vi "iow28_io-ports_write.vi"() -> ()   [LabVIEW 2011]
panel:
  out "Error Read":errorcluster caption="error"
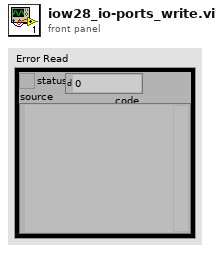
[diagram p1: front panel]
types:
  T1 = typedef "IOWarrior_Handle.ctl" = cluster{"Handle":u32, "Serial Number":string, "type of Warrior":T2, "Root Handle":bool, "Revision":u16}
  T2 = typedef "IOWarrior_Type.ctl" = enum16{"invalid", "IOW24", "IOW40", "IOW56", "IOPV1", "IOPV2", "IOW28"}
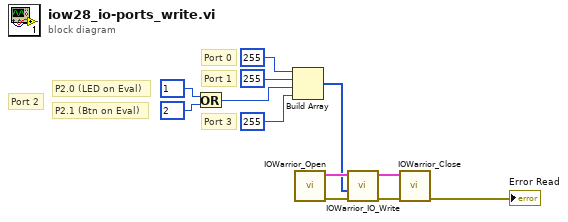
[diagram p0: block diagram]
diagram:
  # "Port 2"
  # "P2.1 (Btn on Eval)"
  # "Port 3"
  # "P2.0 (LED on Eval)"
  # "Port 1"
  # "Port 0"
  n1 = Or(x=u8 1, y=u8 2) -> (x .or. y?=w1:u8)
  n2 = Build Array(u8 255, u8 255, w1, u8 255) -> (w7:u8[])
  n3 = call "IOWarrior_Open.vi"() -> ("err out"=w11:errorcluster, "IOWarriorHandle"=w12:T1)  [unwired: 9 in, 1 out]
  n4 = call "IOWarrior_IO_Write.vi"("err in"=w11, "Array_in"=w7, "devHandle"=w12) -> ("err out"=w10:errorcluster, "devHandleout"=w9:T1)  [unwired: 7 in]
  n5 = call "IOWarrior_Close.vi"("err in"=w10, "devHandle"=w9) -> ("err out"=→"Error Read":errorcluster)  [unwired: 8 in, 1 out]
